vi "Countdown.vi"(11 "String 2":string) -> (3 "String 3":string)   [LabVIEW 2025]
panel:
  out "String":string
  # "GET READY"
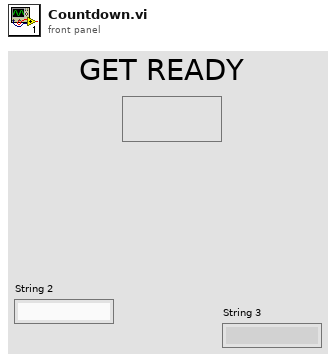
[diagram p1: front panel]
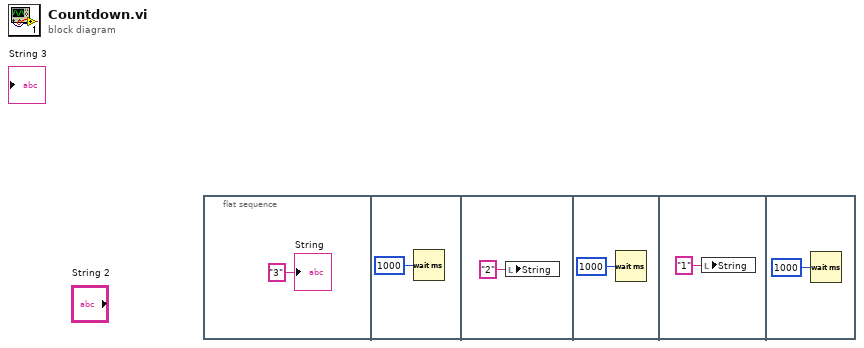
[diagram p0: block diagram]
diagram:
  n1 = flat-sequence {
    frame #0 {
      "String" <- "3" ("String")
    }
    frame #1 {
      n2 = Wait (ms)(milliseconds to wait=u32 1000) -> ()  [unwired: 1 out]
    }
    frame #2 {
      n3 = local write "String"("2" ("String")) -> ()
    }
    frame #3 {
      n4 = Wait (ms)(milliseconds to wait=u32 1000) -> ()  [unwired: 1 out]
    }
    frame #4 {
      n5 = local write "String"("1" ("String")) -> ()
    }
    frame #5 {
      n6 = Wait (ms)(milliseconds to wait=u32 1000) -> ()  [unwired: 1 out]
    }
  }
